vi "Day 15-2.vi"() -> ()   [LabVIEW 2020]
panel:
  out "Min Risk":i32
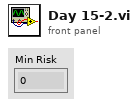
[diagram p1: front panel]
types:
  T1 = typedef "Puzzle 15-1.ctl" = cluster{"Risk":i32[][], "Start":T2, "Goal":T2}
  T2 = typedef "Position.ctl" = cluster{"Row":i32, "Col":i32}
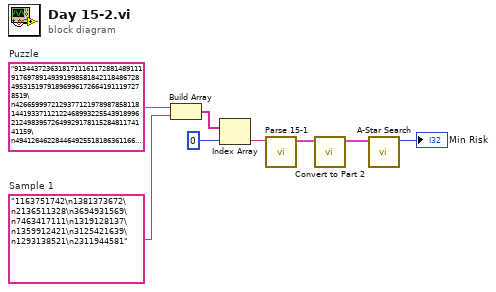
[diagram p0: block diagram]
diagram:
  w7 = "1163751742\n1381373672\n2136511328\n3694931569\n7463417111\n1319128137\n1359912421\n3125421639\n1293138521\n2311944581"  # Sample 1
  w8 = "9134437236318171116117288148911191769789149391998581842118486728495315197918969961726641911197278519\n4266599972129377121978987858118144193371121224689932255439189962124983957264992917811528481174141159\n4941264622844649255181863611661937989592573911314587911782284256729939692285214646949151417873145114\n9945129815342473711424195426247119937972981595714311991417119392838691411867714292812665718171417224\n1423818398213251171691473971673889569992131512132754569226823131415196188491991866258247115715611321\n82719497741914639144311512949281799291721318299439167916189171313423529821826719174729392353297..."  # Puzzle
  n1 = Build Array(w8, w7) -> (w6:string[])
  n2 = Index Array(array=w6, index=0) -> (element=w4:string)
  n3 = call "Parse 15-1.vi"("String"=w4) -> ("Puzzle 15-1"=w2:T1)  [unwired: 10 in]
  n4 = call "Convert to Part 2.vi"("Puzzle 15-1"=w2) -> ("Puzzle 15-2"=w1:T1)  [unwired: 10 in]
  n5 = call "A-Star Search.vi"("Puzzle 15-1 In"=w1) -> ("Min Risk"=→"Min Risk":i32)  [unwired: 10 in]
